vi "UV-VIS GetAcquisitionTimings.vi"(0 "Control in":refnum<class "CCD_camera.lvclass">, 5 "accumulate input":sgl format="%.2f", 7 "kinetic input":sgl format="%.2f", 9 "exposure input":sgl format="%.2f", 11 "error in (no error)":errorcluster) -> (4 "Control out":refnum<class "CCD_camera.lvclass">, 6 "accumulate":sgl format="%.2f", 8 "kinetic":sgl format="%.2f", 10 "DLL error code":u32, 14 "exposure":sgl format="%.2f", 15 "error out":errorcluster)   [LabVIEW 2020, in "CCD_camera.lvclass"]
doc: "This function will return the current \"valid\" acquisition timing information. This function should be used after all the acquisitions settings have been set, e.g. <B>SetExposureTime</B>, <B>SetKineticCycleTime</B> and <B>SetReadMode</B> etc. The values returned are the actual times used in subsequent acquisitions.\n\nThis function is required as it is possible to set the exposure time to 20ms, accumulate cycle time to 30ms and then set the read out mode to full image. As it can take 250ms to read out an image it is not possible to have a cycle time of 30ms.\n\n<B>Parameters:</B>\nexposure - valid exposure time in seconds\naccumulate - valid accumulate cycle time in seconds\nkinetic - valid kinetic cycle time in seconds\n\n<B>Error codes:</B>\nDRV_SUCCESS - Timing information returned.\nDRV_NOT_INITIALIZED - System not initialized.\nDRV_ACQUIRING - Acquisition in progress.\nDRV_INVALID_MODE - Acquisition or readout mode is not available."
uses:
  CCD_camera.lvclass
  C:/dev/TRANCON/Classes/Detector/Detector.lvclass
  Detector.lvclass/Detector.ctl
  Detector.lvclass
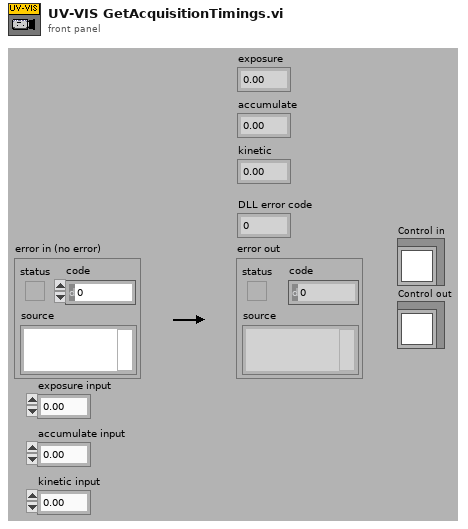
[diagram p1: front panel]
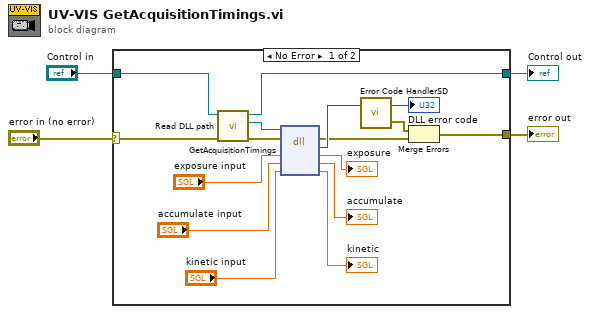
[diagram p0: block diagram]
diagram:
  n1 = case shown="No Error" "error in (no error)" {
    selector: "error in (no error)" -> [w11 w22]
    tunnel: [w6 w22] -> w3
    tunnel: [w5 w21] -> w2
    tunnel: "Control in" -> [w12 w21]
    frame No Error {
      n2 = call "Read DLL path.vi"("error in (no error)"=w11, "Detector in"=w12) -> ("error out"=w10:errorcluster, "DLL path"=w9:path, "Detector out"=w5:refnum<class "CCD_camera.lvclass">)  [unwired: 7 in]
      n3 = dll-call lib="S:/TRANCON/DLL/Atmcd32d.dll" fn="GetAcquisitionTimings"(path in=w9, error in=w10, "exposure"="exposure input", "accumulate"="accumulate input", "kinetic"="kinetic input") -> (error out=w8:errorcluster, "return type"=w20:u32, "exposure"=→"exposure":sgl, "accumulate"=→"accumulate":sgl, "kinetic"=→"kinetic":sgl)  [unwired: 1 in, 1 out]
      n4 = call "Error Code HandlerSD.vi"("DLL error code"=w20) -> ("error out"=w7:errorcluster, "dup DLL error code"=→"DLL error code":u32)  [unwired: 1 in]
      n5 = Merge Errors(w7, w8) -> (w6:errorcluster)
    }
    frame Error {
    }
  }
  "error out" <- w3
  "Control out" <- w2
